vi "Main.vi"(7 "sweep rate, /min":dbl=0.2, 8 "sweep to:":dbl=-0.5, 9 "sweep":T6(radio)=enum."time_sweep") -> ()   [LabVIEW 2017] (continued)
                  tunnel: w2197 -> [w2201 w2205]
                  tunnel: [w2201 w2203] -> w2196
                  frame False {
                    # "not measure 2400 1 current (2400_1_i)"
                  }
                  frame True {
                    w2204 = "2400_1_i"
                    # "measure 2400 1 current (2400_1_i)"
                    n1733 = local read "2400 1 addr"() -> (w2209:u8)
                    n1734 = Number To Decimal String(number=w2209) -> (decimal integer string=w2210:string)  [unwired: 1 in]
                    n1735 = GPIB Clear(3:w2210) -> ()  [unwired: 1 in, 2 out]
                    n1736 = Build Array (concatenate)(w2205, w2204) -> (w2203:string[])
                    n1737 = Concatenate Strings(w2208, w2204, "\t") -> (w2207:string)
                  }
                }
                n1738 = property on="Figure_axis" class="Arr (strict)"("Value"=w2196) -> ()  [unwired: 2 in, 2 out]
                n1739 = property on="data_caption" class="Str"("Value"=w2198) -> ()  [unwired: 2 in, 2 out]
              }
              frame #22 {
                # "2400 2 voltage measure (2400_2_v)"
                n1740 = local read "2400 2 meas v"() -> (w2215:bool)
                n1741 = property on="Figure_axis" class="Arr (strict)"() -> ("Value"=w2212:string[])  [unwired: 2 in, 2 out]
                n1742 = property on="data_caption" class="Str"() -> ("Value"=w2214:string)  [unwired: 2 in, 2 out]
                n1743 = case shown="False" w2215 {
                  tunnel: w2214 -> [w2217 w2223]
                  tunnel: [w2217 w2222] -> w2213
                  tunnel: w2212 -> [w2216 w2220]
                  tunnel: [w2216 w2218] -> w2211
                  frame False {
                    # "not measure 2400 2 voltage (2400_2_v)"
                  }
                  frame True {
                    w2219 = "2400_2_v"
                    # "measure 2400 2 voltage (2400_2_v)"
                    n1744 = local read "2400 2 addr"() -> (w2224:u8)
                    n1745 = Number To Decimal String(number=w2224) -> (decimal integer string=w2225:string)  [unwired: 1 in]
                    n1746 = GPIB Clear(3:w2225) -> ()  [unwired: 1 in, 2 out]
                    n1747 = Build Array (concatenate)(w2220, w2219) -> (w2218:string[])
                    n1748 = Concatenate Strings(w2223, w2219, "\t") -> (w2222:string)
                  }
                }
                n1749 = property on="Figure_axis" class="Arr (strict)"("Value"=w2211) -> ()  [unwired: 2 in, 2 out]
                n1750 = property on="data_caption" class="Str"("Value"=w2213) -> ()  [unwired: 2 in, 2 out]
              }
              frame #23 {
                # "2400 2 current measure (2400_2_i)"
                n1751 = local read "2400 2 meas i"() -> (w2230:bool)
                n1752 = property on="Figure_axis" class="Arr (strict)"() -> ("Value"=w2227:string[])  [unwired: 2 in, 2 out]
                n1753 = property on="data_caption" class="Str"() -> ("Value"=w2229:string)  [unwired: 2 in, 2 out]
                n1754 = case shown="False" w2230 {
                  tunnel: w2229 -> [w2232 w2238]
                  tunnel: [w2232 w2237] -> w2228
                  tunnel: w2227 -> [w2231 w2235]
                  tunnel: [w2231 w2233] -> w2226
                  frame False {
                    # "not measure 2400 2 current (2400_2_i)"
                  }
                  frame True {
                    w2234 = "2400_2_i"
                    # "measure 2400 2 current (2400_2_i)"
                    n1755 = local read "2400 2 addr"() -> (w2239:u8)
                    n1756 = Number To Decimal String(number=w2239) -> (decimal integer string=w2240:string)  [unwired: 1 in]
                    n1757 = GPIB Clear(3:w2240) -> ()  [unwired: 1 in, 2 out]
                    n1758 = Build Array (concatenate)(w2235, w2234) -> (w2233:string[])
                    n1759 = Concatenate Strings(w2238, w2234, "\t") -> (w2237:string)
                  }
                }
                n1760 = property on="Figure_axis" class="Arr (strict)"("Value"=w2226) -> ()  [unwired: 2 in, 2 out]
                n1761 = property on="data_caption" class="Str"("Value"=w2228) -> ()  [unwired: 2 in, 2 out]
              }
              frame #24 {
                # "2400 3 voltage measure (2400_3_v)"
                n1762 = local read "2400 3 meas v"() -> (w2245:bool)
                n1763 = property on="Figure_axis" class="Arr (strict)"() -> ("Value"=w2242:string[])  [unwired: 2 in, 2 out]
                n1764 = property on="data_caption" class="Str"() -> ("Value"=w2244:string)  [unwired: 2 in, 2 out]
                n1765 = case shown="False" w2245 {
                  tunnel: w2244 -> [w2247 w2253]
                  tunnel: [w2247 w2252] -> w2243
                  tunnel: w2242 -> [w2246 w2250]
                  tunnel: [w2246 w2248] -> w2241
                  frame False {
                    # "not measure 2400 3 voltage (2400_3_v)"
                  }
                  frame True {
                    w2249 = "2400_3_v"
                    # "measure 2400 3 voltage (2400_3_v)"
                    n1766 = local read "2400 3 addr"() -> (w2254:u8)
                    n1767 = Number To Decimal String(number=w2254) -> (decimal integer string=w2255:string)  [unwired: 1 in]
                    n1768 = GPIB Clear(3:w2255) -> ()  [unwired: 1 in, 2 out]
                    n1769 = Build Array (concatenate)(w2250, w2249) -> (w2248:string[])
                    n1770 = Concatenate Strings(w2253, w2249, "\t") -> (w2252:string)
                  }
                }
                n1771 = property on="Figure_axis" class="Arr (strict)"("Value"=w2241) -> ()  [unwired: 2 in, 2 out]
                n1772 = property on="data_caption" class="Str"("Value"=w2243) -> ()  [unwired: 2 in, 2 out]
              }
              frame #25 {
                # "2400 3 current measure (2400_3_i)"
                n1773 = local read "2400 3 meas i"() -> (w2260:bool)
                n1774 = property on="Figure_axis" class="Arr (strict)"() -> ("Value"=w2257:string[])  [unwired: 2 in, 2 out]
                n1775 = property on="data_caption" class="Str"() -> ("Value"=w2259:string)  [unwired: 2 in, 2 out]
                n1776 = case shown="True" w2260 {
                  tunnel: w2259 -> [w2262 w2268]
                  tunnel: [w2262 w2267] -> w2258
                  tunnel: w2257 -> [w2261 w2265]
                  tunnel: [w2261 w2263] -> w2256
                  frame False {
                    # "not measure 2400 3 current (2400_3_i)"
                  }
                  frame True {
                    w2264 = "2400_3_i"
                    # "measure 2400 3 current (2400_3_i)"
                    n1777 = local read "2400 3 addr"() -> (w2269:u8)
                    n1778 = Number To Decimal String(number=w2269) -> (decimal integer string=w2270:string)  [unwired: 1 in]
                    n1779 = GPIB Clear(3:w2270) -> ()  [unwired: 1 in, 2 out]
                    n1780 = Build Array (concatenate)(w2265, w2264) -> (w2263:string[])
                    n1781 = Concatenate Strings(w2268, w2264, "\t") -> (w2267:string)
                  }
                }
                n1782 = property on="Figure_axis" class="Arr (strict)"("Value"=w2256) -> ()  [unwired: 2 in, 2 out]
                n1783 = property on="data_caption" class="Str"("Value"=w2258) -> ()  [unwired: 2 in, 2 out]
              }
              frame #26 {
                # "2182A 1 channel 1 measure (2182A_1_ch1)"
                n1784 = local read "2182A 1 ch1"() -> (w2275:bool)
                n1785 = property on="Figure_axis" class="Arr (strict)"() -> ("Value"=w2272:string[])  [unwired: 2 in, 2 out]
                n1786 = property on="data_caption" class="Str"() -> ("Value"=w2274:string)  [unwired: 2 in, 2 out]
                n1787 = case shown="False" w2275 {
                  tunnel: w2274 -> [w2277 w2283]
                  tunnel: [w2277 w2282] -> w2273
                  tunnel: w2272 -> [w2276 w2280]
                  tunnel: [w2276 w2278] -> w2271
                  frame False {
                    # "not measure 2182A 1 channel 1 (2182A_1_ch1)"
                  }
                  frame True {
                    w2279 = "2182A_1_ch1"
                    # "measure 2182A 1 channel 1 (2182A_1_ch1)"
                    n1788 = local read "2182A 1 addr"() -> (w2284:u8)
                    n1789 = Number To Decimal String(number=w2284) -> (decimal integer string=w2285:string)  [unwired: 1 in]
                    n1790 = GPIB Clear(3:w2285) -> ()  [unwired: 1 in, 2 out]
                    n1791 = Build Array (concatenate)(w2280, w2279) -> (w2278:string[])
                    n1792 = Concatenate Strings(w2283, w2279, "\t") -> (w2282:string)
                  }
                }
                n1793 = property on="Figure_axis" class="Arr (strict)"("Value"=w2271) -> ()  [unwired: 2 in, 2 out]
                n1794 = property on="data_caption" class="Str"("Value"=w2273) -> ()  [unwired: 2 in, 2 out]
              }
              frame #27 {
                # "2182A 1 channel 2 measure (2182A_1_ch2)"
                n1795 = local read "2182A 1 ch2"() -> (w2290:bool)
                n1796 = property on="Figure_axis" class="Arr (strict)"() -> ("Value"=w2287:string[])  [unwired: 2 in, 2 out]
                n1797 = property on="data_caption" class="Str"() -> ("Value"=w2289:string)  [unwired: 2 in, 2 out]
                n1798 = case shown="True" w2290 {
                  tunnel: w2289 -> [w2292 w2298]
                  tunnel: [w2292 w2297] -> w2288
                  tunnel: w2287 -> [w2291 w2295]
                  tunnel: [w2291 w2293] -> w2286
                  frame False {
                    # "not measure 2182A 1 channel 2 (2182A_1_ch2)"
                  }
                  frame True {
                    w2294 = "2182A_1_ch2"
                    # "measure 2182A 1 channel 2 (2182A_1_ch2)"
                    n1799 = local read "2182A 1 addr"() -> (w2299:u8)
                    n1800 = Number To Decimal String(number=w2299) -> (decimal integer string=w2300:string)  [unwired: 1 in]
                    n1801 = GPIB Clear(3:w2300) -> ()  [unwired: 1 in, 2 out]
                    n1802 = Build Array (concatenate)(w2295, w2294) -> (w2293:string[])
                    n1803 = Concatenate Strings(w2298, w2294, "\t") -> (w2297:string)
                  }
                }
                n1804 = property on="Figure_axis" class="Arr (strict)"("Value"=w2286) -> ()  [unwired: 2 in, 2 out]
                n1805 = property on="data_caption" class="Str"("Value"=w2288) -> ()  [unwired: 2 in, 2 out]
              }
              frame #28 {
                # "2182A 2 channel 1 measure (2182A_2_ch1)"
                n1806 = local read "2182A 2 ch1"() -> (w2305:bool)
                n1807 = property on="Figure_axis" class="Arr (strict)"() -> ("Value"=w2302:string[])  [unwired: 2 in, 2 out]
                n1808 = property on="data_caption" class="Str"() -> ("Value"=w2304:string)  [unwired: 2 in, 2 out]
                n1809 = case shown="True" w2305 {
                  tunnel: w2304 -> [w2307 w2313]
                  tunnel: [w2307 w2312] -> w2303
                  tunnel: w2302 -> [w2306 w2310]
                  tunnel: [w2306 w2308] -> w2301
                  frame False {
                    # "not measure 2182A 2 channel 1 (2182A_2_ch1)"
                  }
                  frame True {
                    w2309 = "2182A_2_ch1"
                    # "measure 2182A 2 channel 1 (2182A_2_ch1)"
                    n1810 = local read "2182A 2 addr"() -> (w2314:u8)
                    n1811 = Number To Decimal String(number=w2314) -> (decimal integer string=w2315:string)  [unwired: 1 in]
                    n1812 = GPIB Clear(3:w2315) -> ()  [unwired: 1 in, 2 out]
                    n1813 = Build Array (concatenate)(w2310, w2309) -> (w2308:string[])
                    n1814 = Concatenate Strings(w2313, w2309, "\t") -> (w2312:string)
                  }
                }
                n1815 = property on="Figure_axis" class="Arr (strict)"("Value"=w2301) -> ()  [unwired: 2 in, 2 out]
                n1816 = property on="data_caption" class="Str"("Value"=w2303) -> ()  [unwired: 2 in, 2 out]
              }
              frame #29 {
                # "2182A 2 channel 2 measure (2182A_2_ch2)"
                n1817 = local read "2182A 2 ch2"() -> (w2320:bool)
                n1818 = property on="Figure_axis" class="Arr (strict)"() -> ("Value"=w2317:string[])  [unwired: 2 in, 2 out]
                n1819 = property on="data_caption" class="Str"() -> ("Value"=w2319:string)  [unwired: 2 in, 2 out]
                n1820 = case shown="True" w2320 {
                  tunnel: w2319 -> [w2322 w2328]
                  tunnel: [w2322 w2327] -> w2318
                  tunnel: w2317 -> [w2321 w2325]
                  tunnel: [w2321 w2323] -> w2316
                  frame False {
                    # "not measure 2182A 2 channel 2 (2182A_2_ch2)"
                  }
                  frame True {
                    w2324 = "2182A_2_ch2"
                    # "measure 2182A 2 channel 2 (2182A_2_ch2)"
                    n1821 = local read "2182A 2 addr"() -> (w2329:u8)
                    n1822 = Number To Decimal String(number=w2329) -> (decimal integer string=w2330:string)  [unwired: 1 in]
                    n1823 = GPIB Clear(3:w2330) -> ()  [unwired: 1 in, 2 out]
                    n1824 = Build Array (concatenate)(w2325, w2324) -> (w2323:string[])
                    n1825 = Concatenate Strings(w2328, w2324, "\t") -> (w2327:string)
                  }
                }
                n1826 = property on="Figure_axis" class="Arr (strict)"("Value"=w2316) -> ()  [unwired: 2 in, 2 out]
                n1827 = property on="data_caption" class="Str"("Value"=w2318) -> ()  [unwired: 2 in, 2 out]
              }
              frame #30 {
                # "2182A 3 channel 1 measure (2182A_3_ch1)"
                n1828 = local read "2182A 3 ch1"() -> (w2335:bool)
                n1829 = property on="Figure_axis" class="Arr (strict)"() -> ("Value"=w2332:string[])  [unwired: 2 in, 2 out]
                n1830 = property on="data_caption" class="Str"() -> ("Value"=w2334:string)  [unwired: 2 in, 2 out]
                n1831 = case shown="True" w2335 {
                  tunnel: w2334 -> [w2337 w2343]
                  tunnel: [w2337 w2342] -> w2333
                  tunnel: w2332 -> [w2336 w2340]
                  tunnel: [w2336 w2338] -> w2331
                  frame False {
                    # "not measure 2182A 3 channel 1 (2182A_3_ch1)"
                  }
                  frame True {
                    w2339 = "2182A_3_ch1"
                    # "measure 2182A 3 channel 1 (2182A_3_ch1)"
                    n1832 = local read "2182A 3 addr"() -> (w2344:u8)
                    n1833 = Number To Decimal String(number=w2344) -> (decimal integer string=w2345:string)  [unwired: 1 in]
                    n1834 = GPIB Clear(3:w2345) -> ()  [unwired: 1 in, 2 out]
                    n1835 = Build Array (concatenate)(w2340, w2339) -> (w2338:string[])
                    n1836 = Concatenate Strings(w2343, w2339, "\t") -> (w2342:string)
                  }
                }
                n1837 = property on="Figure_axis" class="Arr (strict)"("Value"=w2331) -> ()  [unwired: 2 in, 2 out]
                n1838 = property on="data_caption" class="Str"("Value"=w2333) -> ()  [unwired: 2 in, 2 out]
              }
              frame #31 {
                # "2182A 3 channel 2 measure (2182A_3_ch2)"
                n1839 = local read "2182A 3 ch2"() -> (w2350:bool)
                n1840 = property on="Figure_axis" class="Arr (strict)"() -> ("Value"=w2347:string[])  [unwired: 2 in, 2 out]
                n1841 = property on="data_caption" class="Str"() -> ("Value"=w2349:string)  [unwired: 2 in, 2 out]
                n1842 = case shown="False" w2350 {
                  tunnel: w2349 -> [w2352 w2358]
                  tunnel: [w2352 w2357] -> w2348
                  tunnel: w2347 -> [w2351 w2355]
                  tunnel: [w2351 w2353] -> w2346
                  frame False {
                    # "not measure 2182A 3 channel 2 (2182A_3_ch2)"
                  }
                  frame True {
                    w2354 = "2182A_3_ch2"
                    # "measure 2182A 3 channel 2 (2182A_3_ch2)"
                    n1843 = local read "2182A 3 addr"() -> (w2359:u8)
                    n1844 = Number To Decimal String(number=w2359) -> (decimal integer string=w2360:string)  [unwired: 1 in]
                    n1845 = GPIB Clear(3:w2360) -> ()  [unwired: 1 in, 2 out]
                    n1846 = Build Array (concatenate)(w2355, w2354) -> (w2353:string[])
                    n1847 = Concatenate Strings(w2358, w2354, "\t") -> (w2357:string)
                  }
                }
                n1848 = property on="Figure_axis" class="Arr (strict)"("Value"=w2346) -> ()  [unwired: 2 in, 2 out]
                n1849 = property on="data_caption" class="Str"("Value"=w2348) -> ()  [unwired: 2 in, 2 out]
              }
              frame #32 {
                # "2182A 4 channel 1 measure (2182A_4_ch1)"
                n1850 = local read "2182A 4 ch1"() -> (w2365:bool)
                n1851 = property on="Figure_axis" class="Arr (strict)"() -> ("Value"=w2362:string[])  [unwired: 2 in, 2 out]
                n1852 = property on="data_caption" class="Str"() -> ("Value"=w2364:string)  [unwired: 2 in, 2 out]
                n1853 = case shown="True" w2365 {
                  tunnel: w2364 -> [w2367 w2373]
                  tunnel: [w2367 w2372] -> w2363
                  tunnel: w2362 -> [w2366 w2370]
                  tunnel: [w2366 w2368] -> w2361
                  frame False {
                    # "not measure 2182A 4 channel 1 (2182A_4_ch1)"
                  }
                  frame True {
                    w2369 = "2182A_4_ch1"
                    # "measure 2182A 4 channel 1 (2182A_4_ch1)"
                    n1854 = local read "2182A 4 addr"() -> (w2374:u8)
                    n1855 = Number To Decimal String(number=w2374) -> (decimal integer string=w2375:string)  [unwired: 1 in]
                    n1856 = GPIB Clear(3:w2375) -> ()  [unwired: 1 in, 2 out]
                    n1857 = Build Array (concatenate)(w2370, w2369) -> (w2368:string[])
                    n1858 = Concatenate Strings(w2373, w2369, "\t") -> (w2372:string)
                  }
                }
                n1859 = property on="Figure_axis" class="Arr (strict)"("Value"=w2361) -> ()  [unwired: 2 in, 2 out]
                n1860 = property on="data_caption" class="Str"("Value"=w2363) -> ()  [unwired: 2 in, 2 out]
              }
              frame #33 {
                # "2182A 4 channel 2 measure (2182A_4_ch2)"
                n1861 = local read "2182A 4 ch2"() -> (w2380:bool)
                n1862 = property on="Figure_axis" class="Arr (strict)"() -> ("Value"=w2377:string[])  [unwired: 2 in, 2 out]
                n1863 = property on="data_caption" class="Str"() -> ("Value"=w2379:string)  [unwired: 2 in, 2 out]
                n1864 = case shown="True" w2380 {
                  tunnel: w2379 -> [w2382 w2388]
                  tunnel: [w2382 w2387] -> w2378
                  tunnel: w2377 -> [w2381 w2385]
                  tunnel: [w2381 w2383] -> w2376
                  frame False {
                    # "not measure 2182A 4 channel 2 (2182A_4_ch2)"
                  }
                  frame True {
                    w2384 = "2182A_4_ch2"
                    # "measure 2182A 4 channel 2 (2182A_4_ch2)"
                    n1865 = local read "2182A 4 addr"() -> (w2389:u8)
                    n1866 = Number To Decimal String(number=w2389) -> (decimal integer string=w2390:string)  [unwired: 1 in]
                    n1867 = GPIB Clear(3:w2390) -> ()  [unwired: 1 in, 2 out]
                    n1868 = Build Array (concatenate)(w2385, w2384) -> (w2383:string[])
                    n1869 = Concatenate Strings(w2388, w2384, "\t") -> (w2387:string)
                  }
                }
                n1870 = property on="Figure_axis" class="Arr (strict)"("Value"=w2376) -> ()  [unwired: 2 in, 2 out]
                n1871 = property on="data_caption" class="Str"("Value"=w2378) -> ()  [unwired: 2 in, 2 out]
              }
              frame #34 {
                # "2636A smua measure voltage (2636A_smua_v)"
                n1872 = local read "2636A smua meas v"() -> (w2395:bool)
                n1873 = property on="Figure_axis" class="Arr (strict)"() -> ("Value"=w2392:string[])  [unwired: 2 in, 2 out]
                n1874 = property on="data_caption" class="Str"() -> ("Value"=w2394:string)  [unwired: 2 in, 2 out]
                n1875 = case shown="True" w2395 {
                  tunnel: w2394 -> [w2397 w2408]
                  tunnel: [w2397 w2407] -> w2393
                  tunnel: w2392 -> [w2396 w2405]
                  tunnel: [w2396 w2403] -> w2391
                  frame False {
                    # "not measure voltage on 2636A smua (2636A_smua_v)"
                  }
                  frame True {
                    w2404 = "2636A_smua_v"
                    # "measure voltage on 2636A smua (2636A_smua_v)"
                    n1876 = local read "2336A addr"() -> (w2399:refnum<visa-resource-name>)
                    n1877 = VISA Open(VISA resource name=w2399) -> (VISA resource name=w2398:refnum<visa-resource-name>, error out=w2400:errorcluster)  [unwired: 4 in]
                    n1878 = VISA Clear(VISA resource name=w2398, error in (no error)=w2400) -> (VISA resource name out=w2402:refnum<visa-resource-name>)  [unwired: 1 out]
                    n1879 = property class="Instr"(reference=w2402, "General Settings:Timeout Value"=u32 10000) -> ()  [unwired: 1 in, 2 out]
                    n1880 = Build Array (concatenate)(w2405, w2404) -> (w2403:string[])
                    n1881 = Concatenate Strings(w2408, w2404, "\t") -> (w2407:string)
                  }
                }
                n1882 = property on="Figure_axis" class="Arr (strict)"("Value"=w2391) -> ()  [unwired: 2 in, 2 out]
                n1883 = property on="data_caption" class="Str"("Value"=w2393) -> ()  [unwired: 2 in, 2 out]
              }
              frame #35 {
                # "2636A smua measure current (2636A_smua_i)"
                n1884 = local read "2636A smua meas i"() -> (w2413:bool)
                n1885 = property on="Figure_axis" class="Arr (strict)"() -> ("Value"=w2410:string[])  [unwired: 2 in, 2 out]
                n1886 = property on="data_caption" class="Str"() -> ("Value"=w2412:string)  [unwired: 2 in, 2 out]
                n1887 = case shown="True" w2413 {
                  tunnel: w2412 -> [w2415 w2426]
                  tunnel: [w2415 w2425] -> w2411
                  tunnel: w2410 -> [w2414 w2423]
                  tunnel: [w2414 w2421] -> w2409
                  frame False {
                    # "not measure current on 2636A smua (2636A_smua_i)"
                  }
                  frame True {
                    w2422 = "2636A_smua_i"
                    # "measure current on 2636A smua (2636A_smua_i)"
                    n1888 = local read "2336A addr"() -> (w2418:refnum<visa-resource-name>)
                    n1889 = VISA Open(VISA resource name=w2418) -> (VISA resource name=w2417:refnum<visa-resource-name>, error out=w2416:errorcluster)  [unwired: 4 in]
                    n1890 = VISA Clear(VISA resource name=w2417, error in (no error)=w2416) -> (VISA resource name out=w2419:refnum<visa-resource-name>)  [unwired: 1 out]
                    n1891 = Build Array (concatenate)(w2423, w2422) -> (w2421:string[])
                    n1892 = property class="Instr"(reference=w2419, "General Settings:Timeout Value"=u32 10000) -> ()  [unwired: 1 in, 2 out]
                    n1893 = Concatenate Strings(w2426, w2422, "\t") -> (w2425:string)
                  }
                }
                n1894 = property on="Figure_axis" class="Arr (strict)"("Value"=w2409) -> ()  [unwired: 2 in, 2 out]
                n1895 = property on="data_caption" class="Str"("Value"=w2411) -> ()  [unwired: 2 in, 2 out]
              }
              frame #36 {
                # "2636A smub measure voltage (2636A_smub_v)"
                n1896 = local read "2636A smub meas v"() -> (w2431:bool)
                n1897 = property on="Figure_axis" class="Arr (strict)"() -> ("Value"=w2428:string[])  [unwired: 2 in, 2 out]
                n1898 = property on="data_caption" class="Str"() -> ("Value"=w2430:string)  [unwired: 2 in, 2 out]
                n1899 = case shown="True" w2431 {
                  tunnel: w2430 -> [w2433 w2444]
                  tunnel: [w2433 w2443] -> w2429
                  tunnel: w2428 -> [w2432 w2441]
                  tunnel: [w2432 w2439] -> w2427
                  frame False {
                    # "not measure voltage on 2636A smub (2636A_smub_v)"
                  }
                  frame True {
                    w2440 = "2636A_smub_v"
                    # "measure voltage on 2636A smub (2636A_smub_v)"
                    n1900 = local read "2336A addr"() -> (w2435:refnum<visa-resource-name>)
                    n1901 = VISA Open(VISA resource name=w2435) -> (VISA resource name=w2434:refnum<visa-resource-name>, error out=w2436:errorcluster)  [unwired: 4 in]
                    n1902 = VISA Clear(VISA resource name=w2434, error in (no error)=w2436) -> (VISA resource name out=w2437:refnum<visa-resource-name>)  [unwired: 1 out]
                    n1903 = Build Array (concatenate)(w2441, w2440) -> (w2439:string[])
                    n1904 = property class="Instr"(reference=w2437, "General Settings:Timeout Value"=u32 10000) -> ()  [unwired: 1 in, 2 out]
                    n1905 = Concatenate Strings(w2444, w2440, "\t") -> (w2443:string)
                  }
                }
                n1906 = property on="Figure_axis" class="Arr (strict)"("Value"=w2427) -> ()  [unwired: 2 in, 2 out]
                n1907 = property on="data_caption" class="Str"("Value"=w2429) -> ()  [unwired: 2 in, 2 out]
              }
              frame #37 {
                # "2636A smub measure current (2636A_smub_i)"
                n1908 = local read "2636A smub meas i"() -> (w2449:bool)
                n1909 = property on="Figure_axis" class="Arr (strict)"() -> ("Value"=w2446:string[])  [unwired: 2 in, 2 out]
                n1910 = property on="data_caption" class="Str"() -> ("Value"=w2448:string)  [unwired: 2 in, 2 out]
                n1911 = case shown="True" w2449 {
                  tunnel: w2448 -> [w2451 w2462]
                  tunnel: [w2451 w2461] -> w2447
                  tunnel: w2446 -> [w2450 w2459]
                  tunnel: [w2450 w2457] -> w2445
                  frame False {
                    # "not measure current on 2636A smub (2636A_smub_i)"
                  }
                  frame True {
                    w2458 = "2636A_smub_i"
                    # "measure current on 2636A smub (2636A_smub_i)"
                    n1912 = local read "2336A addr"() -> (w2452:refnum<visa-resource-name>)
                    n1913 = VISA Open(VISA resource name=w2452) -> (VISA resource name=w2453:refnum<visa-resource-name>, error out=w2454:errorcluster)  [unwired: 4 in]
                    n1914 = VISA Clear(VISA resource name=w2453, error in (no error)=w2454) -> (VISA resource name out=w2455:refnum<visa-resource-name>)  [unwired: 1 out]
                    n1915 = Build Array (concatenate)(w2459, w2458) -> (w2457:string[])
                    n1916 = property class="Instr"(reference=w2455, "General Settings:Timeout Value"=u32 10000) -> ()  [unwired: 1 in, 2 out]
                    n1917 = Concatenate Strings(w2462, w2458, "\t") -> (w2461:string)
                  }
                }
                n1918 = property on="Figure_axis" class="Arr (strict)"("Value"=w2445) -> ()  [unwired: 2 in, 2 out]
                n1919 = property on="data_caption" class="Str"("Value"=w2447) -> ()  [unwired: 2 in, 2 out]
              }
              frame #38 {
                # "measure time"
                n1920 = local read "measure time"() -> (w2467:bool)
                n1921 = property on="Figure_axis" class="Arr (strict)"() -> ("Value"=w2464:string[])  [unwired: 2 in, 2 out]
                n1922 = property on="data_caption" class="Str"() -> ("Value"=w2466:string)  [unwired: 2 in, 2 out]
                n1923 = case shown="True" w2467 {
                  tunnel: w2466 -> [w2469 w2475]
                  tunnel: [w2469 w2474] -> w2465
                  tunnel: w2464 -> [w2468 w2472]
                  tunnel: [w2468 w2470] -> w2463
                  frame False {
                    # "not measuring time"
                  }
                  frame True {
                    w2471 = "time"
                    # "measuring time"
                    n1924 = Build Array (concatenate)(w2472, w2471) -> (w2470:string[])
                    n1925 = Concatenate Strings(w2475, w2471, "\t") -> (w2474:string)
                  }
                }
                n1926 = property on="Figure_axis" class="Arr (strict)"("Value"=w2463) -> ()  [unwired: 2 in, 2 out]
                n1927 = property on="data_caption" class="Str"("Value"=w2465) -> ()  [unwired: 2 in, 2 out]
              }
              frame #39 {
                # "Measure magnetic field on IPS120-0"
                n1928 = local read "iPS_MagnetField"() -> (w2480:bool)
                n1929 = property on="Figure_axis" class="Arr (strict)"() -> ("Value"=w2477:string[])  [unwired: 2 in, 2 out]
                n1930 = property on="data_caption" class="Str"() -> ("Value"=w2479:string)  [unwired: 2 in, 2 out]
                n1931 = case shown="True" w2480 {
                  tunnel: w2479 -> [w2482 w2488]
                  tunnel: [w2482 w2487] -> w2478
                  tunnel: w2477 -> [w2481 w2485]
                  tunnel: [w2481 w2483] -> w2476
                  frame False {
                    # "do not Measure magnetic field on IPS120-0"
                  }
                  frame True {
                    w2484 = "iPS_MagntField"
                    n1932 = Build Array (concatenate)(w2485, w2484) -> (w2483:string[])
                    n1933 = Concatenate Strings(w2488, w2484, "\t") -> (w2487:string)
                  }
                }
                n1934 = property on="Figure_axis" class="Arr (strict)"("Value"=w2476) -> ()  [unwired: 2 in, 2 out]
                n1935 = property on="data_caption" class="Str"("Value"=w2478) -> ()  [unwired: 2 in, 2 out]
              }
              frame #40 {
                # "Measure Magnet_T on iPS"
                n1936 = property on="Magnet_T" class="Bool (strict)"() -> ("Value"=w2489:bool)  [unwired: 2 in, 2 out]
                n1937 = property on="Figure_axis" class="Arr (strict)"() -> ("Value"=w2491:string[])  [unwired: 2 in, 2 out]
                n1938 = property on="data_caption" class="Str"() -> ("Value"=w2493:string)  [unwired: 2 in, 2 out]
                n1939 = case shown="True" w2489 {
                  tunnel: w2493 -> [w2495 w2501]
                  tunnel: [w2495 w2500] -> w2492
                  tunnel: w2491 -> [w2494 w2498]
                  tunnel: [w2494 w2496] -> w2490
                  frame False {
                    # "do not Measure magnetic field on IPS120-0"
                  }
                  frame True {
                    w2497 = "iPS_Magnet_T"
                    n1940 = Build Array (concatenate)(w2498, w2497) -> (w2496:string[])
                    n1941 = Concatenate Strings(w2501, w2497, "\t") -> (w2500:string)
                  }
                }
                n1942 = property on="Figure_axis" class="Arr (strict)"("Value"=w2490) -> ()  [unwired: 2 in, 2 out]
                n1943 = property on="data_caption" class="Str"("Value"=w2492) -> ()  [unwired: 2 in, 2 out]
              }
              frame #41 {
                # "Measure SH_T on iPS"
                n1944 = property on="SH_T" class="Bool (strict)"() -> ("Value"=w2502:bool)  [unwired: 2 in, 2 out]
                n1945 = property on="Figure_axis" class="Arr (strict)"() -> ("Value"=w2504:string[])  [unwired: 2 in, 2 out]
                n1946 = property on="data_caption" class="Str"() -> ("Value"=w2506:string)  [unwired: 2 in, 2 out]
                n1947 = case shown="False" w2502 {
                  tunnel: w2506 -> [w2508 w2514]
                  tunnel: [w2508 w2513] -> w2505
                  tunnel: w2504 -> [w2507 w2511]
                  tunnel: [w2507 w2509] -> w2503
                  frame False {
                    # "do not Measure magnetic field on IPS120-0"
                  }
                  frame True {
                    w2510 = "iPS_SH_T"
                    n1948 = Build Array (concatenate)(w2511, w2510) -> (w2509:string[])
                    n1949 = Concatenate Strings(w2514, w2510, "\t") -> (w2513:string)
                  }
                }
                n1950 = property on="Figure_axis" class="Arr (strict)"("Value"=w2503) -> ()  [unwired: 2 in, 2 out]
                n1951 = property on="data_caption" class="Str"("Value"=w2505) -> ()  [unwired: 2 in, 2 out]
              }
              frame #42 {
                # "iTC sample Temp"
                n1952 = property on="iTC_Sample_T" class="Bool (strict)"() -> ("Value"=w2515:bool)  [unwired: 2 in, 2 out]
                n1953 = property on="Figure_axis" class="Arr (strict)"() -> ("Value"=w2517:string[])  [unwired: 2 in, 2 out]
                n1954 = property on="data_caption" class="Str"() -> ("Value"=w2519:string)  [unwired: 2 in, 2 out]
                n1955 = case shown="True" w2515 {
                  tunnel: w2519 -> [w2521 w2527]
                  tunnel: [w2521 w2526] -> w2518
                  tunnel: w2517 -> [w2520 w2524]
                  tunnel: [w2520 w2522] -> w2516
                  frame False {
                    # "not measure 2461 voltage (2461_meas_v)"
                  }
                  frame True {
                    w2523 = "iTC_Sample_T"
                    n1956 = Build Array (concatenate)(w2524, w2523) -> (w2522:string[])
                    n1957 = Concatenate Strings(w2527, w2523, "\t") -> (w2526:string)
                  }
                }
                n1958 = property on="Figure_axis" class="Arr (strict)"("Value"=w2516) -> ()  [unwired: 2 in, 2 out]
                n1959 = property on="data_caption" class="Str"("Value"=w2518) -> ()  [unwired: 2 in, 2 out]
              }
              frame #43 {
                # "iTC sample Temp"
                n1960 = property on="VTI_T" class="Bool (strict)"() -> ("Value"=w2528:bool)  [unwired: 2 in, 2 out]
                n1961 = property on="Figure_axis" class="Arr (strict)"() -> ("Value"=w2530:string[])  [unwired: 2 in, 2 out]
                n1962 = property on="data_caption" class="Str"() -> ("Value"=w2532:string)  [unwired: 2 in, 2 out]
                n1963 = case shown="True" w2528 {
                  tunnel: w2532 -> [w2534 w2540]
                  tunnel: [w2534 w2539] -> w2531
                  tunnel: w2530 -> [w2533 w2537]
                  tunnel: [w2533 w2535] -> w2529
                  frame False {
                    # "not measure 2461 voltage (2461_meas_v)"
                  }
                  frame True {
                    w2536 = "iTC_VTI_T"
                    n1964 = Build Array (concatenate)(w2537, w2536) -> (w2535:string[])
                    n1965 = Concatenate Strings(w2540, w2536, "\t") -> (w2539:string)
                  }
                }
                n1966 = property on="Figure_axis" class="Arr (strict)"("Value"=w2529) -> ()  [unwired: 2 in, 2 out]
                n1967 = property on="data_caption" class="Str"("Value"=w2531) -> ()  [unwired: 2 in, 2 out]
              }
              frame #44 {
                # "iTC sample Temp"
                n1968 = property on="PT1_T" class="Bool (strict)"() -> ("Value"=w2541:bool)  [unwired: 2 in, 2 out]
                n1969 = property on="Figure_axis" class="Arr (strict)"() -> ("Value"=w2543:string[])  [unwired: 2 in, 2 out]
                n1970 = property on="data_caption" class="Str"() -> ("Value"=w2545:string)  [unwired: 2 in, 2 out]
                n1971 = case shown="True" w2541 {
                  tunnel: w2545 -> [w2547 w2553]
                  tunnel: [w2547 w2552] -> w2544
                  tunnel: w2543 -> [w2546 w2550]
                  tunnel: [w2546 w2548] -> w2542
                  frame False {
                    # "not measure 2461 voltage (2461_meas_v)"
                  }
                  frame True {
                    w2549 = "iTC_PT1_T"
                    n1972 = Build Array (concatenate)(w2550, w2549) -> (w2548:string[])
                    n1973 = Concatenate Strings(w2553, w2549, "\t") -> (w2552:string)
                  }
                }
                n1974 = property on="Figure_axis" class="Arr (strict)"("Value"=w2542) -> ()  [unwired: 2 in, 2 out]
                n1975 = property on="data_caption" class="Str"("Value"=w2544) -> ()  [unwired: 2 in, 2 out]
              }
              frame #45 {
                # "iTC sample Temp"
                n1976 = property on="PT2_T" class="Bool (strict)"() -> ("Value"=w2554:bool)  [unwired: 2 in, 2 out]
                n1977 = property on="Figure_axis" class="Arr (strict)"() -> ("Value"=w2556:string[])  [unwired: 2 in, 2 out]
                n1978 = property on="data_caption" class="Str"() -> ("Value"=w2558:string)  [unwired: 2 in, 2 out]
                n1979 = case shown="True" w2554 {
                  tunnel: w2558 -> [w2560 w2566]
                  tunnel: [w2560 w2565] -> w2557
                  tunnel: w2556 -> [w2559 w2563]
                  tunnel: [w2559 w2561] -> w2555
                  frame False {
                    # "not measure 2461 voltage (2461_meas_v)"
                  }
                  frame True {
                    w2562 = "iTC_PT2_T"
                    n1980 = Build Array (concatenate)(w2563, w2562) -> (w2561:string[])
                    n1981 = Concatenate Strings(w2566, w2562, "\t") -> (w2565:string)
                  }
                }
                n1982 = property on="Figure_axis" class="Arr (strict)"("Value"=w2555) -> ()  [unwired: 2 in, 2 out]
                n1983 = property on="data_caption" class="Str"("Value"=w2557) -> ()  [unwired: 2 in, 2 out]
              }
              frame #46 {
                # "iTC sample Temp"
                n1984 = property on="VTI_P" class="Bool (strict)"() -> ("Value"=w2567:bool)  [unwired: 2 in, 2 out]
                n1985 = property on="Figure_axis" class="Arr (strict)"() -> ("Value"=w2569:string[])  [unwired: 2 in, 2 out]
                n1986 = property on="data_caption" class="Str"() -> ("Value"=w2571:string)  [unwired: 2 in, 2 out]
                n1987 = case shown="True" w2567 {
                  tunnel: w2571 -> [w2573 w2579]
                  tunnel: [w2573 w2578] -> w2570
                  tunnel: w2569 -> [w2572 w2576]
                  tunnel: [w2572 w2574] -> w2568
                  frame False {
                    # "not measure 2461 voltage (2461_meas_v)"
                  }
                  frame True {
                    w2575 = "iTC_VTI_P"
                    n1988 = Build Array (concatenate)(w2576, w2575) -> (w2574:string[])
                    n1989 = Concatenate Strings(w2579, w2575, "\t") -> (w2578:string)
                  }
                }
                n1990 = property on="Figure_axis" class="Arr (strict)"("Value"=w2568) -> ()  [unwired: 2 in, 2 out]
                n1991 = property on="data_caption" class="Str"("Value"=w2570) -> ()  [unwired: 2 in, 2 out]
              }
              frame #47 {
                # "iTC sample Temp"
                n1992 = property on="2461_meas_v" class="Bool (strict)"() -> ("Value"=w2580:bool)  [unwired: 2 in, 2 out]
                n1993 = property on="Figure_axis" class="Arr (strict)"() -> ("Value"=w2582:string[])  [unwired: 2 in, 2 out]
                n1994 = property on="data_caption" class="Str"() -> ("Value"=w2584:string)  [unwired: 2 in, 2 out]
                n1995 = case shown="True" w2580 {
                  tunnel: w2584 -> [w2586 w2592]
                  tunnel: [w2586 w2591] -> w2583
                  tunnel: w2582 -> [w2585 w2589]
                  tunnel: [w2585 w2587] -> w2581
                  frame False {
                    # "not measure 2461 voltage (2461_meas_v)"
                  }
                  frame True {
                    w2588 = "2461_meas_v"
                    n1996 = Build Array (concatenate)(w2589, w2588) -> (w2587:string[])
                    n1997 = Concatenate Strings(w2592, w2588, "\t") -> (w2591:string)
                  }
                }
                n1998 = property on="Figure_axis" class="Arr (strict)"("Value"=w2581) -> ()  [unwired: 2 in, 2 out]
                n1999 = property on="data_caption" class="Str"("Value"=w2583) -> ()  [unwired: 2 in, 2 out]
              }
              frame #48 {
                # "iTC sample Temp"
                n2000 = property on="2461_meas_i" class="Bool (strict)"() -> ("Value"=w2593:bool)  [unwired: 2 in, 2 out]
                n2001 = property on="Figure_axis" class="Arr (strict)"() -> ("Value"=w2595:string[])  [unwired: 2 in, 2 out]
                n2002 = property on="data_caption" class="Str"() -> ("Value"=w2597:string)  [unwired: 2 in, 2 out]
                n2003 = case shown="True" w2593 {
                  tunnel: w2597 -> [w2599 w2605]
                  tunnel: [w2599 w2604] -> w2596
                  tunnel: w2595 -> [w2598 w2602]
                  tunnel: [w2598 w2600] -> w2594
                  frame False {
                    # "not measure 2461 voltage (2461_meas_v)"
                  }
                  frame True {
                    w2601 = "2461_meas_i"
                    n2004 = Build Array (concatenate)(w2602, w2601) -> (w2600:string[])
                    n2005 = Concatenate Strings(w2605, w2601, "\t") -> (w2604:string)
                  }
                }
                n2006 = property on="Figure_axis" class="Arr (strict)"("Value"=w2594) -> ()  [unwired: 2 in, 2 out]
                n2007 = property on="data_caption" class="Str"("Value"=w2596) -> ()  [unwired: 2 in, 2 out]
              }
              frame #49 {
                # "iTC sample Temp"
                n2008 = property on="Step Loop" class="Bool (strict)"() -> ("Value"=w2606:bool)  [unwired: 2 in, 2 out]
                n2009 = property on="Figure_axis" class="Arr (strict)"() -> ("Value"=w2608:string[])  [unwired: 2 in, 2 out]
                n2010 = property on="data_caption" class="Str"() -> ("Value"=w2610:string)  [unwired: 2 in, 2 out]
                n2011 = case shown="True" w2606 {
                  tunnel: w2610 -> [w2612 w2621]
                  tunnel: [w2612 w2620] -> w2609
                  tunnel: w2608 -> [w2611 w2618]
                  tunnel: [w2611 w2617] -> w2607
                  frame False {
                    # "not measure 2461 voltage (2461_meas_v)"
                  }
                  frame True {
                    n2012 = property on="step" class="RadioBtnsControl (strict)"() -> ("Value"=w2616:T8)  [unwired: 2 in, 2 out]
                    n2013 = case shown="\"iPS_step\"" w2616 {
                      tunnel: ["V2400_1" "V2400_2" "Va" "Vb" "time" "iTC" "iPS"] -> w2614
                      frame "V2400_1_Step", Default {
                      }
                      frame "V2400_2_step" {
                      }
                      frame "2636_smua_step" {
                      }
                      frame "2636_smub_step" {
                      }
                      frame "time_step" {
                      }
                      frame "iTC_step" {
                      }
                      frame "iPS_step" {
                      }
                    }
                    n2014 = Concatenate Strings(w2614, "_Step") -> (w2613:string)
                    n2015 = Build Array (concatenate)(w2618, w2613) -> (w2617:string[])
                    n2016 = Concatenate Strings(w2621, w2613, "\t") -> (w2620:string)
                  }
                }
                n2017 = property on="Figure_axis" class="Arr (strict)"("Value"=w2607) -> ()  [unwired: 2 in, 2 out]
                n2018 = property on="data_caption" class="Str"("Value"=w2609) -> ()  [unwired: 2 in, 2 out]
              }
              frame #50 {
                # "iTC sample Temp"
                n2019 = property on="HyperLoop" class="Bool (strict)"() -> ("Value"=w2629:bool)  [unwired: 2 in, 2 out]
                n2020 = property on="Figure_axis" class="Arr (strict)"() -> ("Value"=w2631:string[])  [unwired: 2 in, 2 out]
                n2021 = property on="data_caption" class="Str"() -> ("Value"=w2633:string)  [unwired: 2 in, 2 out]
                n2022 = case shown="True" w2629 {
                  tunnel: w2633 -> [w2635 w2644]
                  tunnel: [w2635 w2643] -> w2632
                  tunnel: w2631 -> [w2634 w2641]
                  tunnel: [w2634 w2640] -> w2630
                  frame False {
                    # "not measure 2461 voltage (2461_meas_v)"
                  }
                  frame True {
                    n2023 = property on="step_hyper" class="RadioBtnsControl (strict)"() -> ("Value"=w2639:T9)  [unwired: 2 in, 2 out]
                    n2024 = case shown="\"iPS_HyperLoop\"" w2639 {
                      tunnel: ["V2400_1" "V2400_2" "Va" "Vb" "time" "iTC" "iPS"] -> w2637
                      frame "2400_1_HyperLoop", Default {
                      }
                      frame "2400_2_HyperLoop" {
                      }
                      frame "2636_smua_HyperLoop" {
                      }
                      frame "2636_smub_HyperLoop" {
                      }
                      frame "time_HyperLoop" {
                      }
                      frame "iTC_HyperLoop" {
                      }
                      frame "iPS_HyperLoop" {
                      }
                    }
                    n2025 = Concatenate Strings(w2637, "_HyperLoop") -> (w2636:string)
                    n2026 = Build Array (concatenate)(w2641, w2636) -> (w2640:string[])
                    n2027 = Concatenate Strings(w2644, w2636, "\t") -> (w2643:string)
                  }
                }
                n2028 = property on="Figure_axis" class="Arr (strict)"("Value"=w2630) -> ()  [unwired: 2 in, 2 out]
                n2029 = property on="data_caption" class="Str"("Value"=w2632) -> ()  [unwired: 2 in, 2 out]
              }
              frame #51 {
                # "iTC sample Temp"
                n2030 = property on="SuperHyper" class="Bool (strict)"() -> ("Value"=w2652:bool)  [unwired: 2 in, 2 out]
                n2031 = property on="data_caption" class="Str"() -> ("Value"=w2656:string)  [unwired: 2 in, 2 out]
                n2032 = property on="Figure_axis" class="Arr (strict)"() -> ("Value"=w2654:string[])  [unwired: 2 in, 2 out]
                n2033 = case shown="True" w2652 {
                  tunnel: w2656 -> [w2658 w2667]
                  tunnel: [w2658 w2666] -> w2655
                  tunnel: w2654 -> [w2657 w2664]
                  tunnel: [w2657 w2663] -> w2653
                  frame False {
                    # "not measure 2461 voltage (2461_meas_v)"
                  }
                  frame True {
                    n2034 = property on="step_super" class="RadioBtnsControl (strict)"() -> ("Value"=w2659:T10)  [unwired: 2 in, 2 out]
                    n2035 = case shown="\"iTC_SuperHyper\"" w2659 {
                      tunnel: ["V2400_1" "V2400_2" "Va" "Vb" "time" "iTC" "iPS"] -> w2661
                      frame "2400_1_SuperHyper", Default {
                      }
                      frame "2400_2_SuperHyper" {
                      }
                      frame "2636_smua_SuperHyper" {
                      }
                      frame "2636_smub_SuperHyper" {
                      }
                      frame "time_SuperHyper" {
                      }
                      frame "iTC_SuperHyper" {
                      }
                      frame "iPS_SuperHyper" {
                      }
                    }
                    n2036 = Concatenate Strings(w2661, "_SuperHyper") -> (w2660:string)
                    n2037 = Build Array (concatenate)(w2664, w2660) -> (w2663:string[])
                    n2038 = Concatenate Strings(w2667, w2660, "\t") -> (w2666:string)
                  }
                }
                n2039 = property on="Figure_axis" class="Arr (strict)"("Value"=w2653) -> ()  [unwired: 2 in, 2 out]
                n2040 = property on="data_caption" class="Str"("Value"=w2655) -> ()  [unwired: 2 in, 2 out]
              }
            }
          }
          frame #2 {
            # "1 = 2400 1\n2 = 2400 2\n3 = 2400 3\n4 = 2636a smua\n5 = 2636a smub\n6 = do not sweep, just time\n7 = Teslatron_iPS_Field\n8 = Teslatron_iTC_Sample T"
            n2041 = property on="sweep" class="RadioBtnsControl (strict)"() -> ("Value"=w2675:T6)  [unwired: 2 in, 2 out]
            n2042 = case "reads current value from instrument which will be sweeping" shown="\"iPS\"" w2675 {
              tunnel: [w2677 w2687 w2696 w2705 w2709 0.0 ("Measuremet") w2715 w2735 w2738] -> w2676
              frame "2400_1", Default {
                # "reads the voltage on 2400 1"
                n2043 = local read "2400 1 addr"() -> (w2681:u8)
                n2044 = Number To Decimal String(number=w2681) -> (decimal integer string=w2682:string)  [unwired: 1 in]
                n2045 = GPIB Write(0:w2682, 1:":READ?") -> (6:w2678:errorcluster)  [unwired: 3 in, 1 out]
                n2046 = GPIB Read(0:w2682, 1:3200, 3:w2678) -> (5:w2684:string)  [unwired: 2 in, 2 out]
                n2047 = String Subset(string=w2684, length (rest)=13) -> (substring=w2685:string)  [unwired: 1 in]
                n2048 = Fract/Exp String To Number(string=w2685) -> (number=w2677:dbl)  [unwired: 3 in, 1 out]
              }
              frame "2400_2" {
                # "reads the current on 2400 2"
                n2049 = local read "2400 2 addr"() -> (w2691:u8)
                n2050 = Number To Decimal String(number=w2691) -> (decimal integer string=w2692:string)  [unwired: 1 in]
                n2051 = GPIB Write(0:w2692, 1:":READ?") -> (6:w2688:errorcluster)  [unwired: 3 in, 1 out]
                n2052 = GPIB Read(0:w2692, 1:3200, 3:w2688) -> (5:w2694:string)  [unwired: 2 in, 2 out]
                n2053 = String Subset(string=w2694, offset (0)=14, length (rest)=13) -> (substring=w2695:string)
                n2054 = Fract/Exp String To Number(string=w2695) -> (number=w2687:dbl)  [unwired: 3 in, 1 out]
              }
              frame "2400_3" {
                # "reads the voltage on 2400 3"
                n2055 = local read "2400 3 addr"() -> (w2700:u8)
                n2056 = Number To Decimal String(number=w2700) -> (decimal integer string=w2701:string)  [unwired: 1 in]
                n2057 = GPIB Write(0:w2701, 1:":READ?") -> (6:w2697:errorcluster)  [unwired: 3 in, 1 out]
                n2058 = GPIB Read(0:w2701, 1:3200, 3:w2697) -> (5:w2703:string)  [unwired: 2 in, 2 out]
                n2059 = String Subset(string=w2703, length (rest)=13) -> (substring=w2704:string)  [unwired: 1 in]
                n2060 = Fract/Exp String To Number(string=w2704) -> (number=w2696:dbl)  [unwired: 3 in, 1 out]
              }
              frame "2636a_smua" {
                # "reads the voltage on 2636a smua"
                n2061 = local read "2336A addr"() -> (w2708:refnum<visa-resource-name>)
                n2062 = call "SinglePointMeasurement.vi"("Measure"=Measure."Voltage", "Channel"=Channel."a", "VISA resource name 2"=w2708) -> ("Measuremet"=w2705:dbl)  [unwired: 3 in, 4 out]
              }
              frame "2636a_smub" {
                # "reads the voltage on 2636a smub"
                n2063 = local read "2336A addr"() -> (w2712:refnum<visa-resource-name>)
                n2064 = call "SinglePointMeasurement.vi"("Measure"=Measure."Voltage", "Channel"=Channel."b", "VISA resource name 2"=w2712) -> ("Measuremet"=w2709:dbl)  [unwired: 3 in, 4 out]
              }
              frame "time_sweep" {
              }
              frame "iPS" {
                n2065 = property on="Sweep B" class="Bool (strict)"() -> ("Value"=w2714:bool)  [unwired: 2 in, 2 out]
                n2066 = case shown="False" w2714 {
                  tunnel: [w2716 w2734] -> w2715
                  frame False {
                    n2067 = stacked-sequence {
                      tunnel: [_ _ w2723 _] -> w2716
                      frame #0 {
                        n2068 = local read "iPS_addr_sweep"() -> (w2719:refnum<visa-resource-name>)
                        n2069 = property on="sweep to:" class="DigNum (strict)"() -> ("Value"=w2717:dbl)  [unwired: 2 in, 2 out]
                        n2070 = call "iPSset.vi"("Target Field, T"=w2717, "iPSSetCtrl"=iPSsetCtrl."Set Target Field", "VISA resource name"=w2719) -> ()  [unwired: 5 in, 4 out]
                      }
                      frame #1 {
                        n2071 = local read "iPS_addr_sweep"() -> (w2722:refnum<visa-resource-name>)
                        n2072 = property on="sweep rate, /min" class="DigNum (strict)"() -> ("Value"=w2720:dbl)  [unwired: 2 in, 2 out]
                        n2073 = call "iPSset.vi"("Field Rate, T/min"=w2720, "iPSSetCtrl"=iPSsetCtrl."Set Target Field Rate", "VISA resource name"=w2722) -> ()  [unwired: 5 in, 4 out]
                      }
                      frame #2 {
                        n2074 = property on="iPS_addr_sweep" class="VISAName"() -> ("Value"=w2725:refnum<visa-resource-name>)  [unwired: 2 in, 2 out]
                        n2075 = call "iPSread.vi"("iPSreadCtrl"=iPSreadCtrl."OutputField", "VISA resource name"=w2725) -> ("number"=w2723:dbl)  [unwired: 6 in, 3 out]
                      }
                      frame #3 {
                        n2076 = property on="sweep to:" class="DigNum (strict)"() -> ("Value"=w2726:dbl)  [unwired: 2 in, 2 out]
                        n2077 = Not Equal To 0?(x=w2726) -> (x != 0?=w2729:bool)
                        n2078 = local read "iPS_addr_sweep"() -> (w2731:refnum<visa-resource-name>)
                        n2079 = Select(t=iPSsetCtrl."Go to Field" ("iPSSetCtrl"), s=w2729, f=iPSsetCtrl."Go to Field" ("iPSSetCtrl")) -> (s? t:f=w2727:T18)
                        n2080 = call "iPSset.vi"("iPSSetCtrl"=w2727, "VISA resource name"=w2731) -> ()  [unwired: 6 in, 4 out]
                      }
                    }
                  }
                  frame True {
                    # "Measure magnetic field on IPS120-0"
                    n2081 = property on="iPS_addr_sweep" class="VISAName"() -> ("Value"=w2733:refnum<visa-resource-name>)  [unwired: 2 in, 2 out]
                    n2082 = call "iPSread.vi"("iPSreadCtrl"=iPSreadCtrl."OutputField", "VISA resource name"=w2733) -> ("number"=w2734:dbl)  [unwired: 6 in, 3 out]
                  }
                }
              }
              frame "iTC" {
                n2083 = property on="iTC_addr_sweep" class="VISAName"() -> ("Value"=w2737:refnum<visa-resource-name>)  [unwired: 2 in, 2 out]
                n2084 = call "iTCread.vi"("VISA resource name"=w2737, "iTCreadCtrl"=iTCreadCtrl."Sample Temp") -> ("number"=w2735:dbl)  [unwired: 5 in, 3 out]
              }
              frame "2461" {
                n2085 = property on="2461_addr_sweep" class="VISAName"() -> ("Value"=w2739:refnum<visa-resource-name>)  [unwired: 2 in, 2 out]
                n2086 = call <instrlib>:"Get Source Level.vi"("VISA resource name"=w2739) -> ("Current Level Out"=w2738:dbl)  [unwired: 7 in, 3 out]
              }
            }
          }
          frame #3 {
            n2087 = property on="Step Loop" class="Bool (strict)"() -> ("Value"=w2740:bool)  [unwired: 2 in, 2 out]
            n2088 = case shown="False" w2740 {
              frame False {
                # "Reserve a name for new linetrace data file:"
                n2089 = property on="Data Folder" class="Path"() -> ("Value"=w2748:path)  [unwired: 2 in, 2 out]
                n2090 = call "AutoNamerDatExtraArtem.vi"("SweepType"="linetraces", "Custom User Path"=w2748) -> ("String"=w2746:string, "Path"=w2747:path)  [unwired: 2 in]
                n2091 = Path To String(path=w2747) -> (string=w2745:string)
                n2092 = Concatenate Strings(w2745, "\\", w2746) -> (w2744:string)
                n2093 = String To Path(string=w2744) -> (path=w2743:path)
                n2094 = local write "Data file:"(w2743) -> ()
              }
              frame True {
                n2095 = property on="Sweep Direction" class="Str"() -> ("Value"=w2749:string)  [unwired: 2 in, 2 out]
                n2096 = case shown="\"Sweep Down\"" w2749 {
                  frame "Sweep Up" {
                    n2097 = property on="UpNameString" class="Str"() -> ("Value"=w2751:string)  [unwired: 2 in, 2 out]
                    n2098 = String To Path(string=w2751) -> (path=w2750:path)
                    n2099 = local write "Data file:"(w2750) -> ()
                  }
                  frame "Sweep Down" {
                    n2100 = property on="DownNameString" class="Str"() -> ("Value"=w2752:string)  [unwired: 2 in, 2 out]
                    n2101 = String To Path(string=w2752) -> (path=w2753:path)
                    n2102 = local write "Data file:"(w2753) -> ()
                  }
                  frame "Ramp Down", Default {
                  }
                }
              }
            }
          }
          frame #4 {
            # "add \"formula\" string to the axis rings"
            n2103 = property on="Figure_axis" class="Arr (strict)"() -> ("Value"=w2756:string[])  [unwired: 2 in, 2 out]
            n2104 = Build Array (concatenate)(w2756, "formula") -> (w2754:string[])
            n2105 = property on="Figure_axis" class="Arr (strict)"("Value"=w2754) -> ()  [unwired: 2 in, 2 out]
          }
          frame #5 {
            # "passes array to ring"
            n2106 = property on="SuperHyper" class="Bool (strict)"() -> ("Value"=w2757:bool)  [unwired: 2 in, 2 out]
            n2107 = case shown="False" w2757 {
              frame True {
                # "records the fist line into the both upa nd down data file\nwhen table index=0"
                n2108 = property on="Table Index" class="DigNum (strict)"() -> ("Value"=w2766:dbl)  [unwired: 2 in, 2 out]
                n2109 = property on="HyperLoop Index" class="DigNum (strict)"() -> ("Value"=w2767:dbl)  [unwired: 2 in, 2 out]
                n2110 = property on="SuperHyper_Index" class="DigNum (strict)"() -> ("Value"=w2761:dbl)  [unwired: 2 in, 2 out]
                n2111 = Equal To 0?(x=w2766) -> (x = 0?=w2764:bool)
                n2112 = Equal To 0?(x=w2767) -> (x = 0?=w2765:bool)
                n2113 = Equal To 0?(x=w2761) -> (x = 0?=w2760:bool)
                n2114 = And(x=w2765, y=w2764) -> (x .and. y?=w2763:bool)
                n2115 = And(x=w2763, y=w2760) -> (x .and. y?=w2762:bool)
                n2116 = case shown="True" w2762 {
                  frame False {
                  }
                  frame True {
                    n2117 = property on="data_caption" class="Str"() -> ("Value"=w2771:string)  [unwired: 2 in, 2 out]
                    n2118 = local read "Data file:"() -> (w2768:path)
                    n2119 = Concatenate Strings(w2771, "\r") -> (w2770:string)
                    n2120 = Write to Text File(file (use dialog)=w2768, text=w2770) -> ()  [unwired: 2 in, 3 out]
                  }
                }
              }
              frame False {
                n2121 = property on="HyperLoop" class="Bool (strict)"() -> ("Value"=w2772:bool)  [unwired: 2 in, 2 out]
                n2122 = case shown="False" w2772 {
                  frame False {
                    n2123 = property on="Step Loop" class="Bool (strict)"() -> ("Value"=w2773:bool)  [unwired: 2 in, 2 out]
                    n2124 = case shown="True" w2773 {
                      frame False {
                        # "records the fist line into the data file"
